vi "Return Cmd Notifier.vi"(8 "error in":errorcluster, 9 "Input Data":variant, 10 "Return Data":variant) -> (0 "error out":errorcluster)   [LabVIEW 2012, in "Cmd Queue.lvlib"]
uses:
  Cmd Queue.lvlib
panel:
  out "found":bool
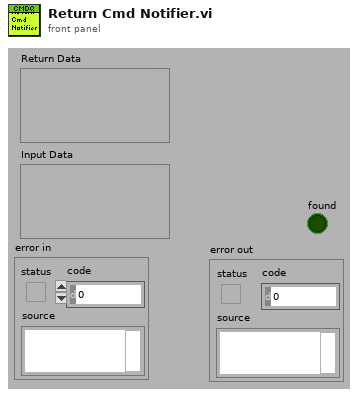
[diagram p1: front panel]
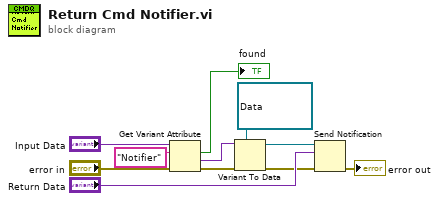
[diagram p0: block diagram]
diagram:
  n1 = Get Variant Attribute(Variant="Input Data", name="Notifier", error in="error in") -> (found=→"found":bool, value=w8:variant, error out=w3:errorcluster)  [unwired: 1 in, 1 out]
  n2 = Variant To Data(error in=w3, type=refnum<notifier> refnum ("notifier out"), Variant=w8) -> (data=w7:refnum<notifier>, error out=w2:errorcluster)
  n3 = Send Notification(notification="Return Data", notifier=w7, error in (no error)=w2) -> (error out=→"error out":errorcluster)  [unwired: 1 out]
